vi "Flatten.vi"(8 "error in (no error)":errorcluster, 11 "Msg in":refnum<class "Msg.lvclass">) -> (0 "error out":errorcluster, 2 "Buffer":u8[](array[numeric]) format="%.0x", 3 "Msg out":refnum<class "Msg.lvclass">)   [LabVIEW 2023, in "ConstellationCommand.lvlib" / "Msg.lvclass"]
uses:
  Msg.lvclass
  Msg.lvclass/Msg.ctl
  ConstellationCommand.lvlib
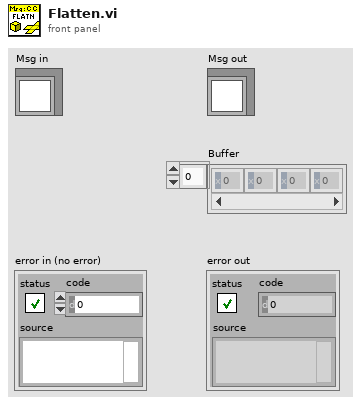
[diagram p1: front panel]
types:
  T1 = typedef "ConstellationCommand.lvlib/Data.ctl" = cluster{"Target Module":string, "Command":string, "Data":string[], "Time Stamp":timestamp}
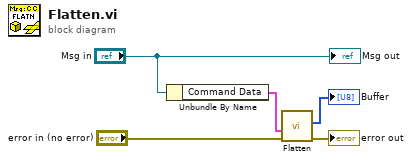
[diagram p0: block diagram]
diagram:
  n1 = Unbundle By Name("Msg in") -> ("Command Data"=w2:T1)
  n2 = call "Flatten.vi"("error in"="error in (no error)", "Command Data"=w2) -> ("error out"=→"error out":errorcluster, "Buffer"=→"Buffer":u8[])  [unwired: 8 in]
  "Msg out" <- "Msg in"
